vi "UpdateROIOffset.vi"(8 "error in (no error)":errorcluster, 9 "ROI Offset Y":dbl, 10 "ROI Offset X":dbl, 11 "Prime95BCameraController in":refnum<class "CameraController.lvclass">) -> (0 "error out":errorcluster, 3 "Prime95BCameraController out":refnum<class "CameraController.lvclass">)   [LabVIEW 2020, in "CameraController.lvlib" / "CameraController.lvclass"]
uses:
  CameraController.lvclass
  CameraController.lvclass/CameraController.ctl
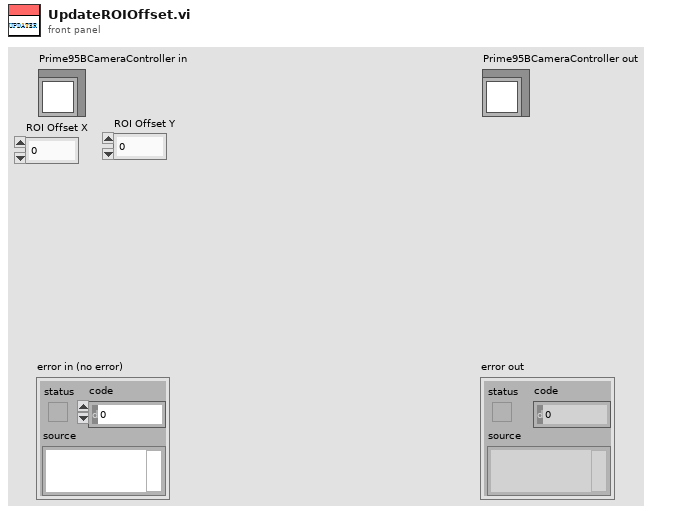
[diagram p1: front panel]
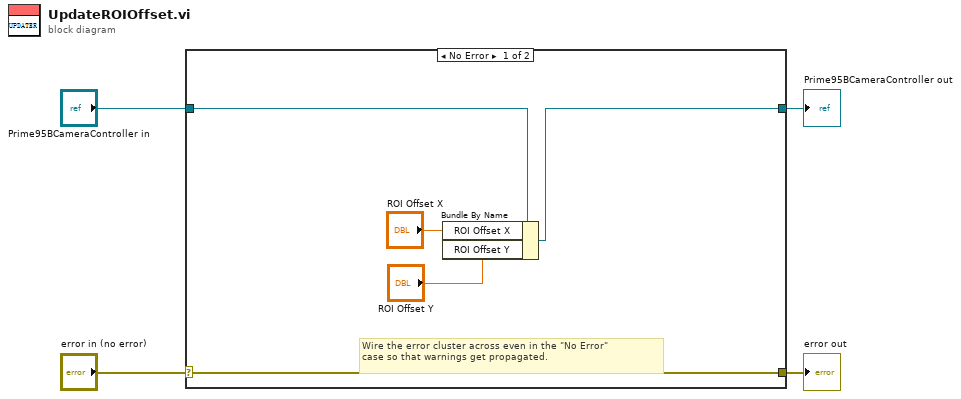
[diagram p0: block diagram]
diagram:
  n1 = case shown="No Error" "error in (no error)" {
    selector: "error in (no error)" -> [w9 w11]
    tunnel: [w9 w11] -> w3
    tunnel: [w7 w10] -> w1
    tunnel: "Prime95BCameraController in" -> [w8 w10]
    frame No Error {
      # "Wire the error cluster across even in the \"No Error\"\ncase so that warnings get propagated."
      n2 = Bundle By Name(cluster=w8, "ROI Offset X"="ROI Offset X", "ROI Offset Y"="ROI Offset Y") -> (w7:refnum<class "CameraController.lvclass">)
    }
    frame Error {
    }
  }
  "error out" <- w3
  "Prime95BCameraController out" <- w1
